vi "Cache.TestSteps.Fglb.vi"(5 "SystemIdx":i32, 7 "Action (get)":T14=enum."get", 8 "error in (no error)":errorcluster, 9 "Result in":T1, 10 "Test in":T6 {"TS"."TP"."value" format="%#.3f"; "TS"."TV"."minimum" format="%#.3f"; "TS"."TV"."maximum" format="%#.3f"}, 11 "Variant":string) -> (0 "error out":errorcluster, 1 "Result out":T1, 2 "Test out":T6 {"TS"."TP"."value" format="%#.3f"; "TS"."TV"."minimum" format="%#.3f"; "TS"."TV"."maximum" format="%#.3f"}, 4 "Found":bool)   [LabVIEW 2016]
uses:
  Cache.TestSteps.Fglb.Action.ctl
  Cache.TestSteps.Fglb.ResultData.ctl
  Database/ProdaNG/Controls/ProdaNG.ProcessResult.ctl
  Database/ProdaNG/Controls/ProdaNG.ProcessStepResult.ctl
  Database/ProdaNG/Controls/ProdaNG.TestStepResult.ctl
  Database/ProdaNG/Controls/ProdaNG.TestValueResult.ctl
  Cache.TestSteps.Fglb.TestData.ctl
  Database/ProdaNG/Controls/ProdaNG.Process.ctl
  Database/ProdaNG/Controls/ProdaNG.ProcessStep.ctl
  Database/ProdaNG/Controls/ProdaNG.ProcessStepParam.ctl
  Database/ProdaNG/Controls/ProdaNG.TestStep.ctl
  Database/ProdaNG/Controls/ProdaNG.TestValue.ctl
  Database/ProdaNG/Controls/ProdaNG.TestStepParam.ctl
  Database/ProdaNG/Controls/ProdaNG.Unit.ctl
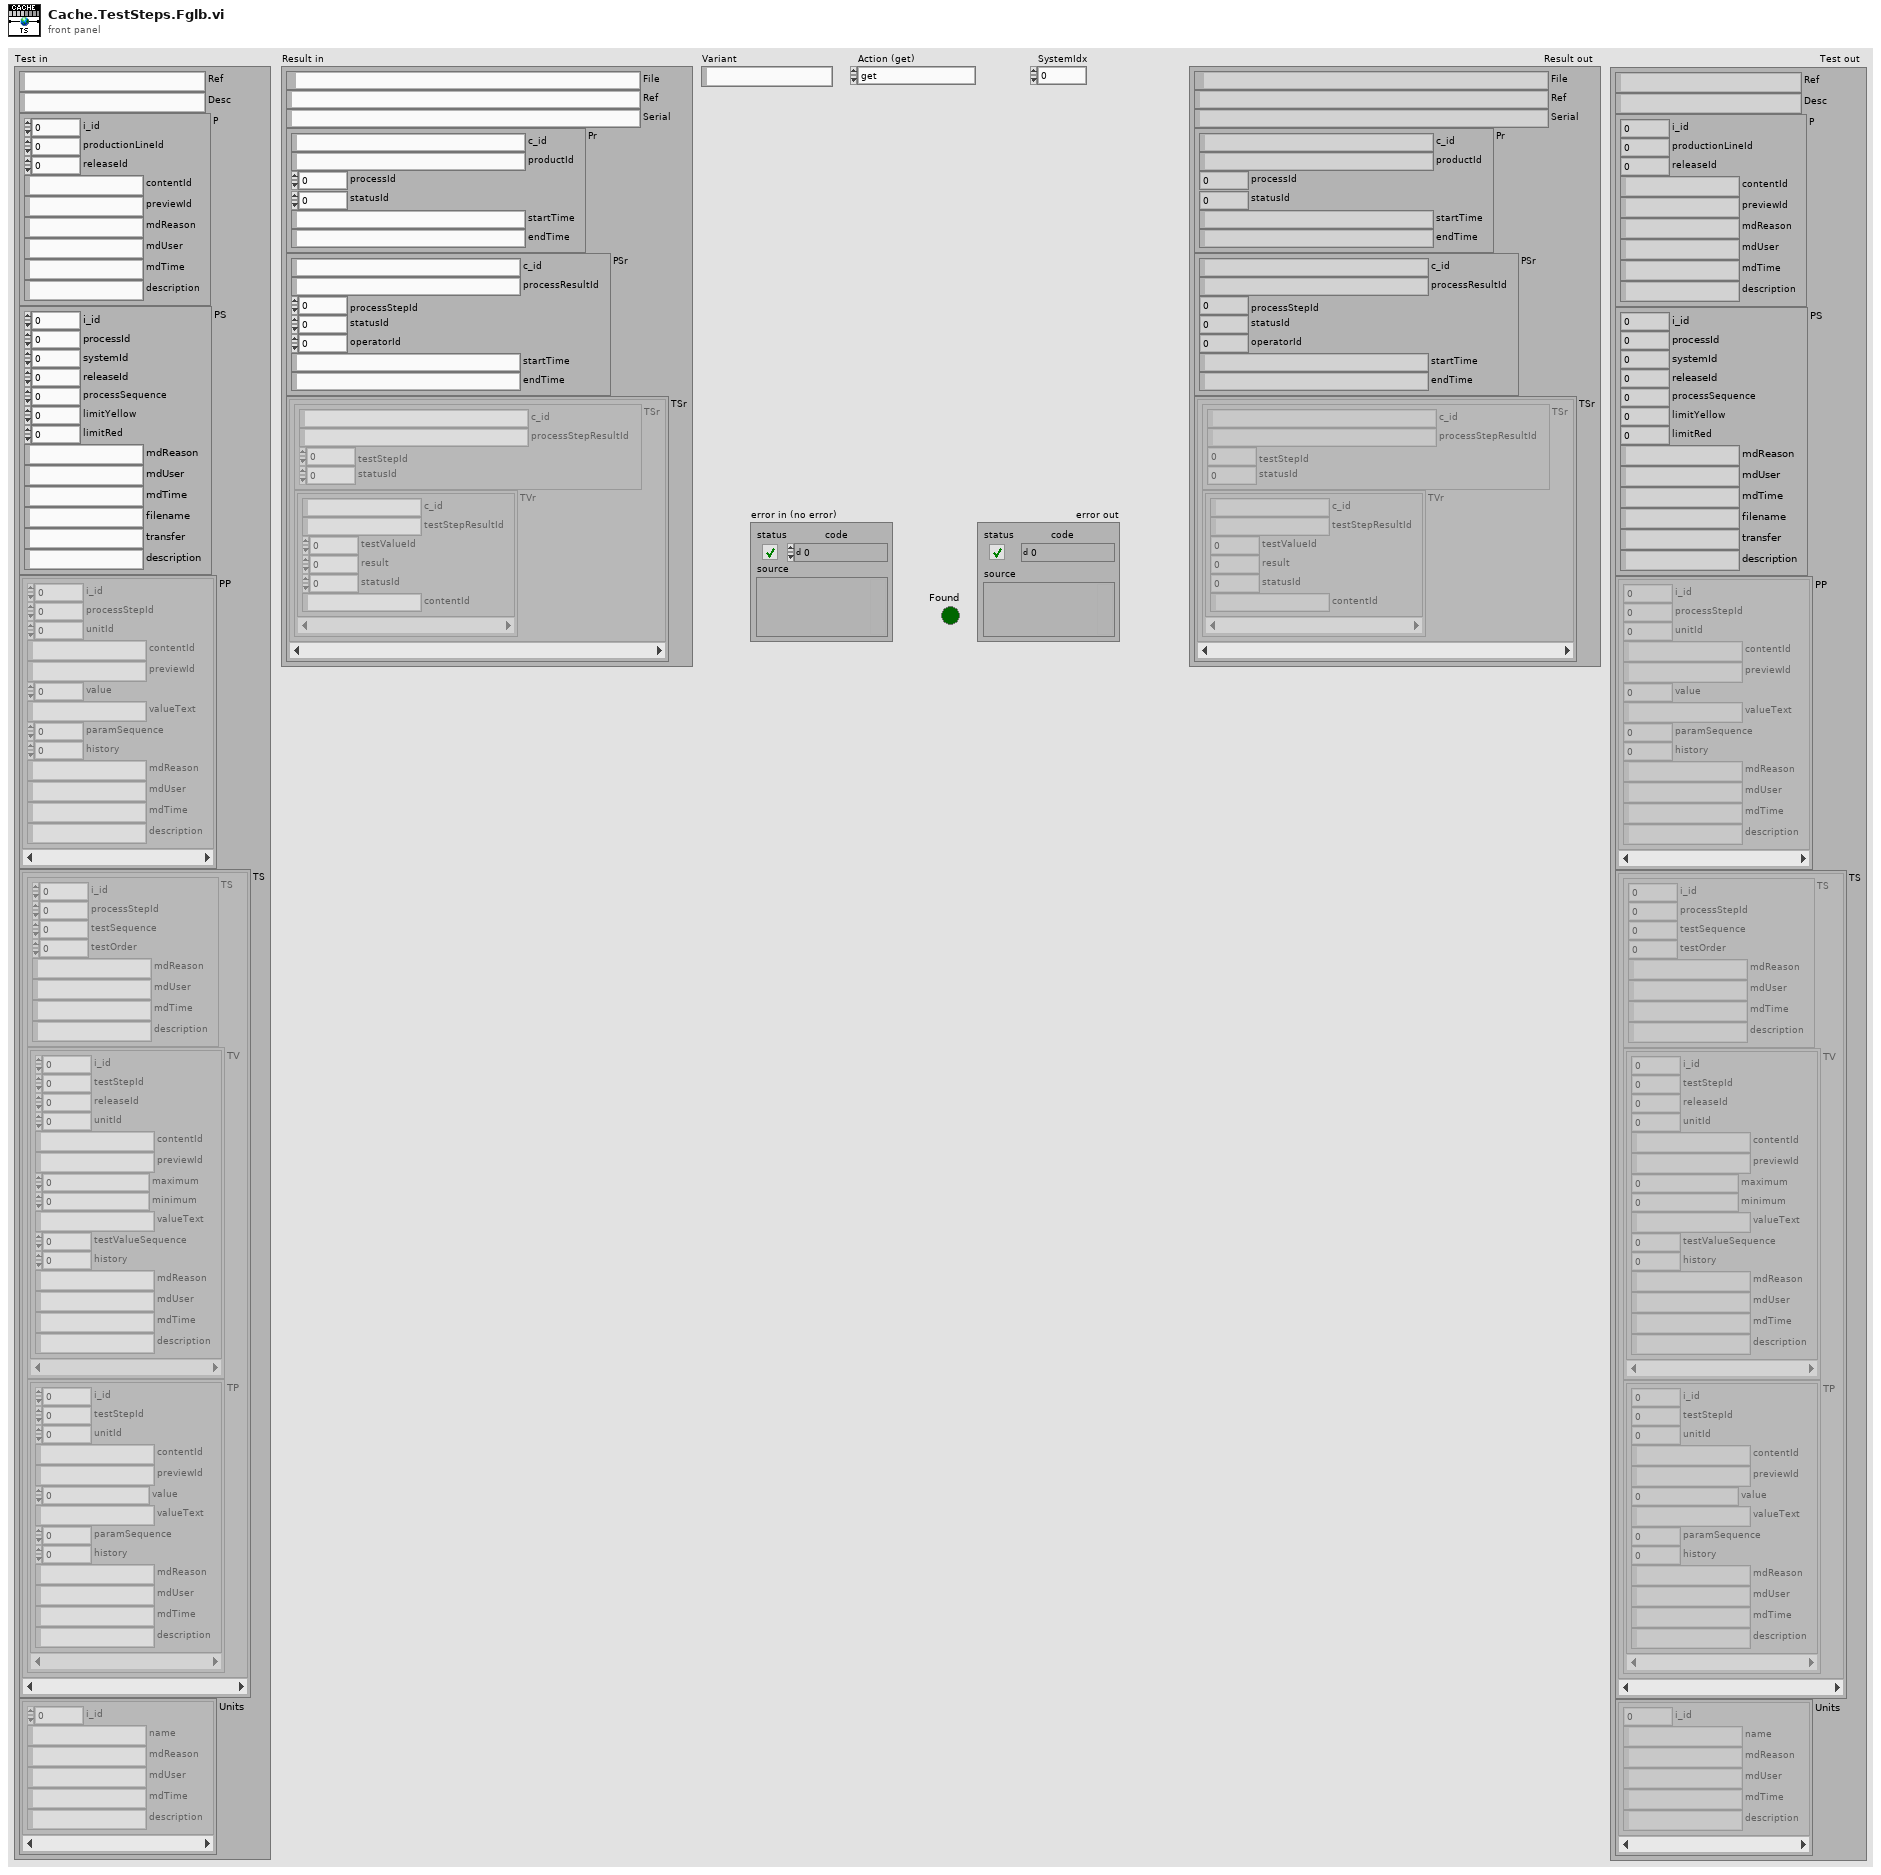
[diagram p1: front panel]
types:
  T1 = typedef "Cache.TestSteps.Fglb.ResultData.ctl" = cluster{"File":path, "Ref":string, "Serial":string, "Pr":T2, "PSr":T3, "TSr":cluster{"TSr":T4, "TVr":T5[]}[]}
  T2 = typedef "ProdaNG.ProcessResult.ctl" = cluster{"c_id":string, "productId":string, "processId":i32, "statusId":i32, "startTime":string, "endTime":string}
  T3 = typedef "ProdaNG.ProcessStepResult.ctl" = cluster{"c_id":string, "processResultId":string, "processStepId":i32, "statusId":i32, "operatorId":i32, "startTime":string, "endTime":string}
  T4 = typedef "ProdaNG.TestStepResult.ctl" = cluster{"c_id":string, "processStepResultId":string, "testStepId":i32, "statusId":i32}
  T5 = typedef "ProdaNG.TestValueResult.ctl" = cluster{"c_id":string, "testStepResultId":string, "testValueId":i32, "result":dbl, "statusId":i32, "contentId":string}
  T6 = typedef "Cache.TestSteps.Fglb.TestData.ctl" = cluster{"Ref":string, "Desc":string, "P":T7, "PS":T8, "PP":T9[], "TS":cluster{"TS":T10, "TV":T11[], "TP":T12[]}[], "Units":T13[]}
  T7 = typedef "ProdaNG.Process.ctl" = cluster{"i_id":i32, "productionLineId":i32, "releaseId":i32, "contentId":string, "previewId":string, "mdReason":string, "mdUser":string, "mdTime":string, "description":string}
  T8 = typedef "ProdaNG.ProcessStep.ctl" = cluster{"i_id":i32, "processId":i32, "systemId":i32, "releaseId":i32, "processSequence":i32, "limitYellow":dbl, "limitRed":dbl, "mdReason":string, "mdUser":string, "mdTime":string, "filename":string, "transfer":string, "description":string}
  T9 = typedef "ProdaNG.ProcessStepParam.ctl" = cluster{"i_id":i32, "processStepId":i32, "unitId":i32, "contentId":string, "previewId":string, "value":dbl, "valueText":string, "paramSequence":i32, "history":i32, "mdReason":string, "mdUser":string, "mdTime":string, "description":string}
  T10 = typedef "ProdaNG.TestStep.ctl" = cluster{"i_id":i32, "processStepId":i32, "testSequence":i32, "testOrder":i32, "mdReason":string, "mdUser":string, "mdTime":string, "description":string}
  T11 = typedef "ProdaNG.TestValue.ctl" = cluster{"i_id":i32, "testStepId":i32, "releaseId":i32, "unitId":i32, "contentId":string, "previewId":string, "maximum":dbl, "minimum":dbl, "valueText":string, "testValueSequence":i32, "history":i32, "mdReason":string, "mdUser":string, "mdTime":string, "description":string}
  T12 = typedef "ProdaNG.TestStepParam.ctl" = cluster{"i_id":i32, "testStepId":i32, "unitId":i32, "contentId":string, "previewId":string, "value":dbl, "valueText":string, "paramSequence":i32, "history":i32, "mdReason":string, "mdUser":string, "mdTime":string, "description":string}
  T13 = typedef "ProdaNG.Unit.ctl" = cluster{"i_id":i32, "name":string, "mdReason":string, "mdUser":string, "mdTime":string, "description":string}
  T14 = typedef "Cache.TestSteps.Fglb.Action.ctl" = enum16{"init", "add", "get"}
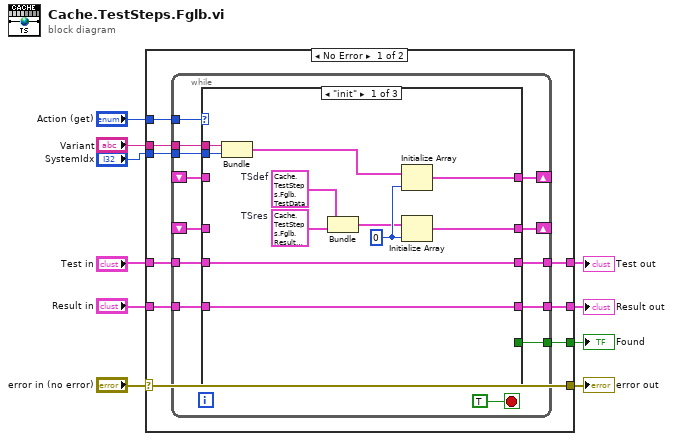
[diagram p0: block diagram]
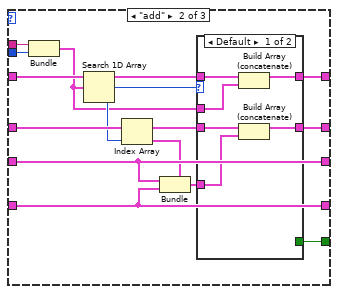
[diagram p2: hidden frame]
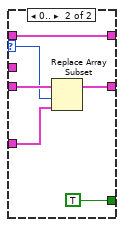
[diagram p3: hidden frame]
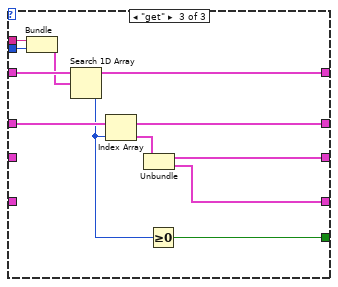
[diagram p4: hidden frame]
diagram:
  n1 = case shown="No Error" "error in (no error)" {
    selector: "error in (no error)" -> [w18 w81]
    tunnel: [w18 w81] -> w9
    tunnel: "Test in" -> [w16 w80]
    tunnel: "Action (get)" -> [w17 _]
    tunnel: "Variant" -> [w19 _]
    tunnel: [w15 w80] -> w3
    tunnel: [w14 _] -> w6
    tunnel: "Result in" -> [w13 w79]
    tunnel: [w12 w79] -> w2
    tunnel: "SystemIdx" -> [w11 _]
    frame No Error {
      n2 = while {
        tunnel: w19 -> [w29]
        tunnel: w17 -> [w32]
        shift-right: [w31] -> _
        shift-left: _ -> [w30]
        shift-right: [w28] -> _
        shift-left: _ -> [w27]
        tunnel: w16 -> [w26]
        tunnel: [w24] -> w15
        tunnel: [w23] -> w14
        tunnel: w13 -> [w22]
        tunnel: [w21] -> w12
        tunnel: w11 -> [w20]
        stop <- TRUE stop-if-true
        n3 = case shown="\"init\"" w32 {
          tunnel: [w39 w55 w78] -> w31
          tunnel: w30 -> [_ w56 w78]
          tunnel: w29 -> [w36 w46 w72]
          tunnel: [w38 w54 w77] -> w28
          tunnel: w27 -> [_ w53 w77]
          tunnel: w26 -> [w42 w49 _]
          tunnel: [w42 w49 w74] -> w24
          tunnel: [_ w52 w76] -> w23
          tunnel: w22 -> [w41 w48 _]
          tunnel: [w41 w48 w69] -> w21
          tunnel: w20 -> [w35 w45 w71]
          frame "init" {
            w40 = 0 ("dimension size")
            w34 = T1 {"File"=path "", "Ref"="", "Serial"="", "Pr"={"c_id"="", "productId"="", "processId"=0, "statusId"=0, "startTime"="", "endTime"=""}, "PSr"={"c_id"="", "processResultId"="", "processStepId"=0, "statusId"=0, "operatorId"=0, "startTime"="", "endTime"=""}, "TSr"=[]}  # TSres
            w43 = T6 {"Ref"="", "Desc"="", "P"={"i_id"=0, "productionLineId"=0, "releaseId"=0, "contentId"="", "previewId"="", "mdReason"="", "mdUser"="", "mdTime"="", "description"=""}, "PS"={"i_id"=0, "processId"=0, "systemId"=0, "releaseId"=0, "processSequence"=0, "limitYellow"=0.0, "limitRed"=0.0, "mdReason"="", "mdUser"="", "mdTime"="", "filename"="", "transfer"="", "description"=""}, "PP"=[], "TS"=[], "Units"=[]}  # TSdef
            n4 = Bundle("Variant"=w36, "SystemIdx"=w35) -> (w33:cluster{"Variant":string, "SystemIdx":i32})  [unwired: 1 in]
            n5 = Bundle("TSdef"=w43, "TSres"=w34) -> (w37:cluster{"TSdef":T6, "TSres":T1})  [unwired: 1 in]
            n6 = Initialize Array(w33, w40) -> (w39:cluster{"Variant":string, "SystemIdx":i32}[])
            n7 = Initialize Array(w37, w40) -> (w38:cluster{"TSdef":T6, "TSres":T1}[])
          }
          frame "add" {
            n8 = Bundle("Variant"=w46, "SystemIdx"=w45) -> (w44:cluster{"Variant":string, "SystemIdx":i32})  [unwired: 1 in]
            n9 = Search 1D Array(1D array=w56, element=w44) -> (index of element=w51:i32)  [unwired: 1 in]
            n10 = Index Array(array=w53, index=w51) -> (element=w47:cluster{"Test in":T6, "Result in":T1})
            n11 = Bundle(cluster=w47, "Test in"=w49, "Result in"=w48) -> (w50:cluster{"Test in":T6, "Result in":T1})
            n12 = case shown="Default" w51 {
              selector: w51 -> [_ w64]
              tunnel: w56 -> [w62 w68]
              tunnel: w53 -> [w60 w67]
              tunnel: w44 -> [w57 _]
              tunnel: [w61 w68] -> w55
              tunnel: [w59 w66] -> w54
              tunnel: [_ TRUE] -> w52
              tunnel: w50 -> [w58 w63]
              frame Default {
                n13 = Build Array (concatenate)(w62, w57) -> (w61:cluster{"Variant":string, "SystemIdx":i32}[])
                n14 = Build Array (concatenate)(w60, w58) -> (w59:cluster{"Test in":T6, "Result in":T1}[])
              }
              frame 0.. {
                n15 = Replace Array Subset(array=w67, new element=w63, index=w64) -> (w66:cluster{"Test in":T6, "Result in":T1}[])
              }
            }
          }
          frame "get" {
            n16 = Bundle("Variant"=w72, "SystemIdx"=w71) -> (w70:cluster{"Variant":string, "SystemIdx":i32})  [unwired: 1 in]
            n17 = Search 1D Array(1D array=w78, element=w70) -> (index of element=w75:i32)  [unwired: 1 in]
            n18 = Index Array(array=w77, index=w75) -> (element=w73:cluster{"Test in":T6, "Result in":T1})
            n19 = Unbundle(w73) -> ("Test in"=w74:T6, "Result in"=w69:T1)
            n20 = Greater Or Equal To 0?(x=w75) -> (x >= 0?=w76:bool)
          }
        }
      }
    }
    frame Error {
    }
  }
  "error out" <- w9
  "Found" <- w6
  "Test out" <- w3
  "Result out" <- w2
